vi "Handshake.vi"(8 "error in (no error)":errorcluster, 9 "timeout ms (5000)":i32=5000, 11 "WebSocket Connection in":refnum<class "WebSocket Server.lvclass">) -> (0 "error out":errorcluster, 3 "WebSocket Connection out":refnum<class "WebSocket Server.lvclass">)   [LabVIEW 2021, in "WebSockets.lvlib" / "WebSocket Server.lvclass"]
doc: "Performs the Server Handshake - reads incoming HTTP WebSocket header from the client and sends the HTTP server response.\nWebSockets 2.0.1.40\nSam Sharp - MediaMongrels Ltd\nCopyright (c) 2019, MediaMongrels Ltd"
uses:
  WebSocket Server.lvclass
  D:/my_projects/projects/Algorithms/Labview/21/WebSockets/WebSockets/WebSocket/WebSocket.lvclass
  WebSocket/WebSocket.lvclass
panel:
  out "HTTP Headers":string
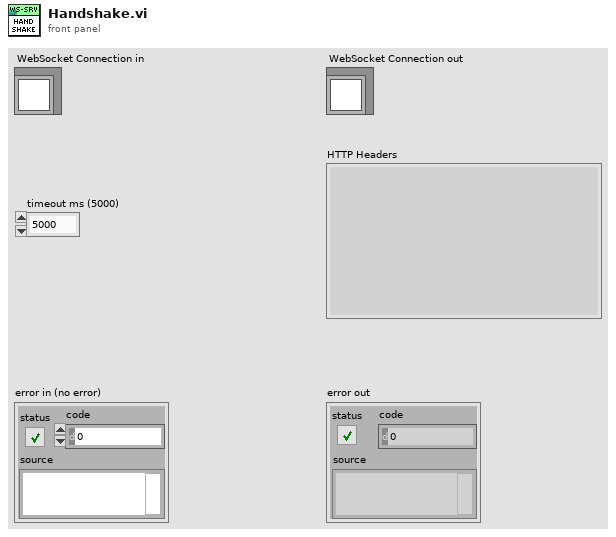
[diagram p1: front panel]
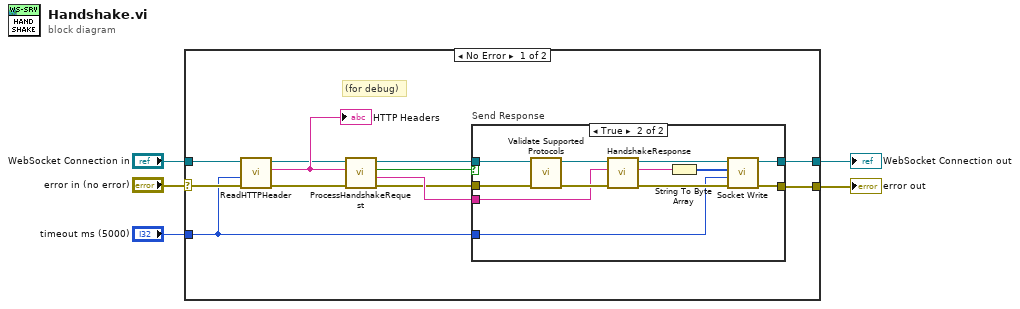
[diagram p0: block diagram]
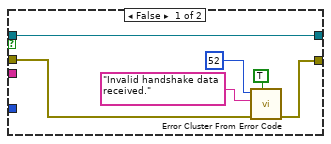
[diagram p2: hidden frame]
diagram:
  n1 = case shown="No Error" "error in (no error)" {
    selector: "error in (no error)" -> [w15 w37]
    tunnel: [w9 w36] -> w5
    tunnel: "WebSocket Connection in" -> [w7 w36]
    tunnel: [w13 w37] -> w2
    tunnel: "timeout ms (5000)" -> [w6 _]
    frame No Error {
      # "(for debug)"
      n2 = call "ReadHTTPHeader.vi"("error in (no error)"=w15, "timeout ms (25000)"=w6, "WebSocket in"=w7) -> ("error out"=w14:errorcluster, "HTTP Header"=w10:string, "WebSocket out"=w8:refnum<class "WebSocket Server.lvclass">)  [unwired: 6 in]
      "HTTP Headers" <- w10
      n3 = call "ProcessHandshakeRequest.vi"("error in (no error)"=w14, "HTTP Header"=w10, "WebSocket in"=w8) -> ("error out"=w16:errorcluster, "Sec-WebSocket-Key"=w17:string, "Is Websocket Request?"=w12:bool, "WebSocket out"=w11:refnum<class "WebSocket Server.lvclass">)  [unwired: 4 in, 1 out]
      n4 = case "Send Response" shown="True" w12 {
        tunnel: w17 -> [_ w24]
        tunnel: w16 -> [w22 w35]
        tunnel: [w23 w26] -> w13
        tunnel: w6 -> [_ w25]
        tunnel: w11 -> [w18 w33]
        tunnel: [w18 w29] -> w9
        frame False {
          n5 = call <vilib>:"Error Cluster From Error Code.vi"("show call chain? (False)"=TRUE, "error in (no error)"=w22, "error message (\"\")"="Invalid handshake data received." ("error message (\"\")"), "error code (0)"=52) -> ("error out"=w23:errorcluster)  [unwired: 5 in]
        }
        frame True {
          n6 = call "Validate Supported Protocols.vi"("error in (no error)"=w35, "WebSocket In"=w33) -> ("error out"=w34:errorcluster, "WebSocket out"=w31:refnum<class "WebSocket Server.lvclass">)  [unwired: 8 in]
          n7 = call "HandshakeResponse.vi"("error in (no error)"=w34, "Sec-WebSocket-Key"=w24, "WebSocket In"=w31) -> ("error out"=w27:errorcluster, "Response Headers"=w32:string, "WebSocket out"=w30:refnum<class "WebSocket Server.lvclass">)  [unwired: 6 in]
          n8 = String To Byte Array(string=w32) -> (unsigned byte array=w28:u8[])
          n9 = call "Socket Write.vi"("error in (no error)"=w27, "timeout ms (5000)"=w25, "Bytes to write"=w28, "WebSocket in"=w30) -> ("error out"=w26:errorcluster, "WebSocket out"=w29:refnum<class "WebSocket Server.lvclass">)  [unwired: 5 in, 1 out]
        }
      }
    }
    frame Error {
    }
  }
  "WebSocket Connection out" <- w5
  "error out" <- w2
